vi "Control Motor.vi"() -> ()   [LabVIEW 2014]
uses:
  <vilib>/LabVIEW Interface for Arduino/Type Defs/Pin Mode.ctl
  <vilib>/LabVIEW Interface for Arduino/LabVIEW Interface for Arduino.lvlib
panel:
  in  "VISA resource":refnum<visa-resource-name>
  in  "stop":bool
  out "Waveform Chart":dbl(graph)
  out "Light Intensity (0 - 100)":dbl(knob) scale=0.0..100.0
  in  "Photo Cell Pin (0)":u8
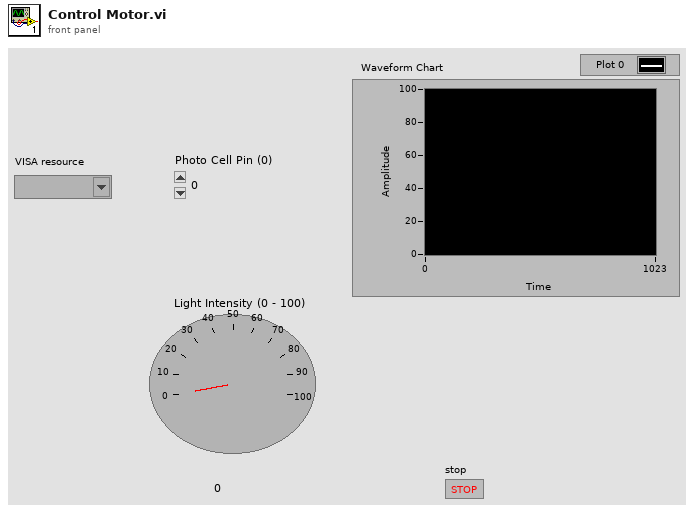
[diagram p1: front panel]
types:
  T1 = typedef "LabVIEW Interface for Arduino.lvlib/Arduino Resource.ctl" = cluster{"VISA resource":refnum<visa-resource-name>, "Board Type":T2, "Connection Type":enum8{"USB / Serial"}, "Bytes Per Packet (15)":u8}
  T2 = typedef "LabVIEW Interface for Arduino.lvlib/Board Type.ctl" = enum16{"Uno", "Dimuelanove w/Atmega 328", "Mega 2560"}
  T3 = typedef "LabVIEW Interface for Arduino.lvlib/Pin Mode.ctl" = enum8{"Input", "Output"}
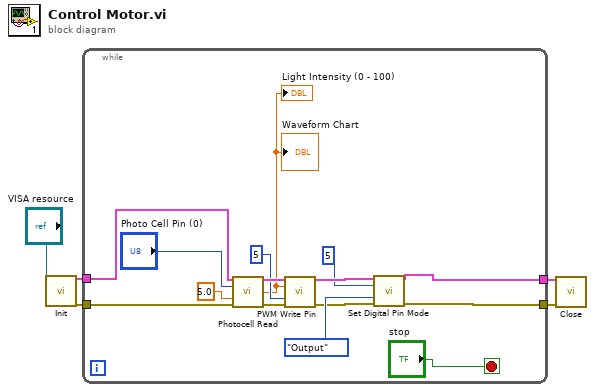
[diagram p0: block diagram]
diagram:
  n1 = call <vilib>:"Init.vi"("VISA resource"="VISA resource") -> ("Arduino Resource"=w5:T1, "error out"=w2:errorcluster)  [unwired: 17 in]
  n2 = while {
    tunnel: w5 -> [w14]
    tunnel: [w7] -> w4
    tunnel: [w6] -> w3
    tunnel: w2 -> [w11]
    stop <- "stop" stop-if-true
    n3 = call <vilib>:"Photocell Read.vi"("Arduino Resource"=w14, "Photo Cell Pin (0)"="Photo Cell Pin (0)", "Vcc (5)"=5.0, "error in"=w11) -> ("Arduino Resource"=w16:T1, "Light Intensity (0 - 100)"=w8:dbl, "error out"=w17:errorcluster)  [unwired: 9 in]
    "Light Intensity (0 - 100)" <- w8
    "Waveform Chart" <- w8
    n4 = call <vilib>:"PWM Write Pin.vi"("Arduino Resource"=w16, "Duty Cycle (0 - 255)"=w8, "PWM Pin (3)"=u8 5, "error in"=w17) -> ("Arduino Resource"=w13:T1, "error out"=w12:errorcluster)  [unwired: 10 in]
    n5 = call <vilib>:"Set Digital Pin Mode.vi"("Arduino Resource"=w13, "Digital I/O Pin"=u8 5, "Pin Mode (Input)"=Pin_Mode."Output", "error in"=w12) -> ("Arduino Resource"=w7:T1, "error out"=w6:errorcluster)  [unwired: 10 in]
  }
  n6 = call <vilib>:"Close.vi"("Arduino Resource"=w4, "error in"=w3) -> ()  [unwired: 13 in, 1 out]
